vi "To Variant.vi"(0 "Derived in":refnum<class "KDemoDerived.lvclass">, 11 "error in (no error)":errorcluster) -> (4 "Derived out":refnum<class "KDemoDerived.lvclass">, 8 "Array":variant[](array[variant]), 15 "error out":errorcluster)   [LabVIEW 2015, in "KDemoDerived.lvclass"]
uses:
  KDemoDerived.lvclass
  KDemoDerived.lvclass/KDemoDerived.ctl
  KDemoBase Class/KDemoBase.lvclass
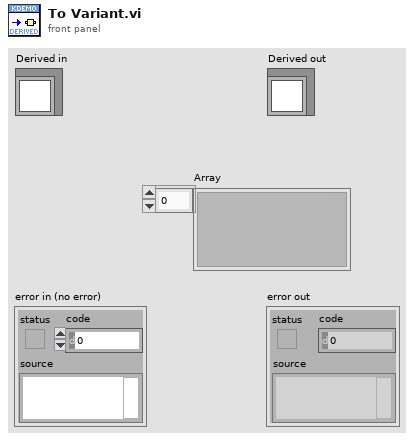
[diagram p1: front panel]
types:
  T1 = typedef "KDemoDerived.lvclass/Serialized.ctl" = cluster{"Integer":i32, "String":string}
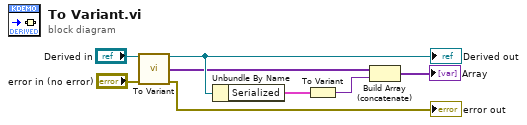
[diagram p0: block diagram]
diagram:
  n1 = call-parent "To Variant.vi"("Base in"="Derived in", "error in (no error)"="error in (no error)") -> ("Base out"=w6:refnum<class "KDemoDerived.lvclass">, "Array"=w4:variant[], "error out"=→"error out":errorcluster)  [unwired: 11 in]
  "Derived out" <- w6
  n2 = Unbundle By Name(w6) -> ("Serialized"=w5:T1)
  n3 = To Variant(anything=w5) -> (Variant=w3:variant)
  n4 = Build Array (concatenate)(w4, w3) -> (→"Array":variant[])
